vi "CompareResponse.vi"(1 "Response":string, 2 "Number":string) -> (0 "Not Equal":bool)   [LabVIEW 2015]
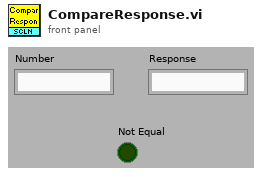
[diagram p1: front panel]
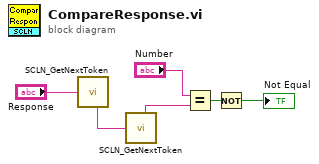
[diagram p0: block diagram]
diagram:
  n1 = call "SCLN_GetNextToken.vi"("Input string"="Response") -> ("Output string"=w5:string)  [unwired: 4 in, 1 out]
  n2 = call "SCLN_GetNextToken.vi"("Input string"=w5) -> ("Token"=w3:string)  [unwired: 4 in, 1 out]
  n3 = Equal?(x="Number", y=w3) -> (x = y?=w2:bool)
  n4 = Not(x=w2) -> (.not. x?=→"Not Equal":bool)
